vi "PH_PILS.vis extExpKnob.vi"(0 "i ref in":refnum<vi>, 5 "error IO":errorcluster) -> (14 "i ref out":refnum<vi>, 19 "error out":errorcluster)   [LabVIEW 2014, in "PH_PILS.lvlib"]
uses:
  PH_PILS.lvlib
  PH_Basics/PH_Common/PH_Common.lvlib
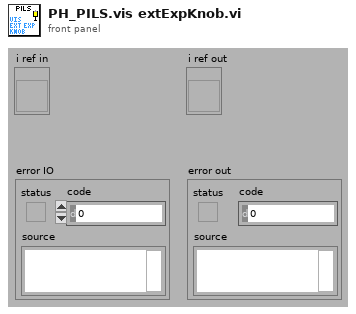
[diagram p1: front panel]
types:
  T1 = typedef "PH_PILS.lvlib/PH_PILS.i attribute.ctl" = cluster{"Boolean":cluster{"GUI Ref":refnum<vi>, "Status":i32}[], "GUI Refs Exp. Shutters":cluster{"1":refnum<vi>, "2":refnum<vi>, "3":refnum<vi>, "4":refnum<vi>}, "Tristate2Run GUI Refs":refnum<vi>[], "EO-Likes":cluster{"GUI Ref":refnum<vi>, "Status":i32}[], "Operation Mode":cluster{"Operation Mode":T2, "GUI":cluster{"Ref State":refnum<vi>, "Ref":refnum<vi>}, "Servicemode":cluster{"Tagname":string, "Status":i32}, "Labormode":cluster{"Tagname":string, "Status":i32}, "Searchmode":cluster{"Tagname":string, "Status":i32}, "Shotmode":cluster{"Tagname":string, "Status":i32}}, "Submode":cluster{"Submode":T3, "GUI":cluster{"Ref State":refnum<vi>, "Ref":refnum<vi>}, "Submode":cluster{"Tagname":string, "Status":i32}}, "Experiment":cluster{"Experiment":enum16{"unknown", "intern", "4 (Z6)", "3", "2", "1"}, "GUI":cluster{"Ref State":refnum<vi>, "Ref":refnum<vi>}, "intern":cluster{"Tagname":string, "Status":i32}, "Exp 4":cluster{"Tagname":string, "Status":i32}, "Exp 3":cluster{"Tagname":string, "Status":i32}, "Exp 2":cluster{"Tagname":string, "Status":i32}, "Exp 1":cluster{"Tagname":string, "Status":i32}}, "TristateNormal":cluster{"GUI Ref":refnum<vi>, "Status":i32}[], "Door Tags":cluster{"GUI Ref":refnum<vi>, "Status":i32}[], "GUIlessTags":cluster{"Name":string, "Status":i32}[], "Beamline GUI Refs":refnum<vi>[], "Special Boolean":cluster{"GUI Ref":refnum<vi>, "Status":i32}[], "Laserpower":cluster{"GUI Ref":refnum<vi>, "Status":i32}[], "Shutter":cluster{"GUI Ref":refnum<vi>, "Status":i32}[], "Tristate EO Like":cluster{"GUI Ref":refnum<vi>, "Status":i32}[], "PP":cluster{"GUI Ref":refnum<vi>, "Status":i32, "Head Ref":refnum<vi>, "Slider Ref":refnum<vi>}[], "Switch Knobs":cluster{"GUI Ref":refnum<vi>, "Status":i32}[], "Latch Knob GUI Refs":refnum<vi>[], "FailureCounter":i32, "Enabled Status":cluster{"Laser":i32, "PreAmp":i32, "MainAmp":i32}, "Mercury":refnum<vi>, "Instance Rods":string, "Logfile":path, "Beckhoff-Instance Internal":string, "Beckhoff-Instance External":string, "Enabling Rights":cluster{"Name":string, "Password":string, "PA?":bool, "MA?":bool, "Exp?":bool}[]}
  T2 = typedef "PH_PILS.lvlib/PH_PILS.Operation Mode.ctl" = enum16{"unknown", "Service", "Labor", "Search", "Shot"}
  T3 = typedef "PH_PILS.lvlib/PH_PILS.Submode.ctl" = enum16{"unknown", "HV-Normal", "HV-Test"}
  T4 = enum16{"unknown", "intern", "4 (Z6)", "3", "2", "1"}
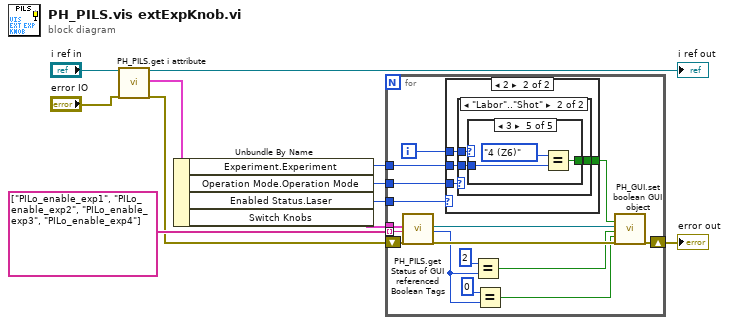
[diagram p0: block diagram]
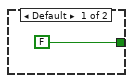
[diagram p2: hidden frame]
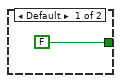
[diagram p3: hidden frame]
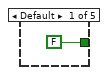
[diagram p4: hidden frame]
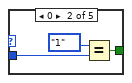
[diagram p5: hidden frame]
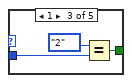
[diagram p6: hidden frame]
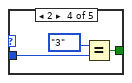
[diagram p7: hidden frame]
diagram:
  n1 = call "PH_PILS.get i attribute.vi"("i ref in"="i ref in", "error in (no error)"="error IO") -> ("i ref out"=→"i ref out":refnum<vi>, "i attribute"=w6:T1, "error out"=w1:errorcluster)  [unwired: 15 in]
  n2 = Unbundle By Name(w6) -> ("Experiment.Experiment"=w5:T4, "Operation Mode.Operation Mode"=w4:T2, "Enabled Status.Laser"=w3:i32, "Switch Knobs"=w7:cluster{"GUI Ref":refnum<vi>, "Status":i32}[])
  n3 = for {
    tunnel: w7 -> [w27]
    tunnel: string[] ["PILo_enable_exp1", "PILo_enable_exp2", "PILo_enable_exp3", "PILo_enable_exp4"] -> [w20] mode=indexing
    tunnel: w5 -> [w18]
    tunnel: w4 -> [w16]
    tunnel: w3 -> [w12]
    shift-right: [w24] -> w11
    shift-left: w1 -> [w23]
    i -> [w19]
    n4 = call "PH_PILS.get Status of GUI referenced Boolean Tags.vi"("Tags"=w27, "Tagname"=w20, "error in"=w23) -> ("GUI Ref"=w25:refnum<vi>, "Status"=w15:i32, "error out"=w26:errorcluster)  [unwired: 13 in, 1 out]
    n5 = case shown="2" w12 {
      tunnel: w19 -> [_ w32]
      tunnel: w18 -> [_ w31]
      tunnel: [FALSE w30] -> w17
      tunnel: w16 -> [_ w29]
      frame Default {
      }
      frame 2 {
        n6 = case shown="\"Labor\"..\"Shot\"" w29 {
          tunnel: w32 -> [_ w36]
          tunnel: w31 -> [_ w35]
          tunnel: [FALSE w34] -> w30
          frame Default {
          }
          frame "Labor".."Shot" {
            n7 = case shown="3" w36 {
              tunnel: w35 -> [_ w39 w42 w45 w48]
              tunnel: [FALSE w38 w41 w44 w47] -> w34
              frame Default {
              }
              frame 0 {
                n8 = Equal?(x=T4."1" ("Experiment.Experiment"), y=w39) -> (x = y?=w38:bool)
              }
              frame 1 {
                n9 = Equal?(x=T4."2" ("Experiment.Experiment"), y=w42) -> (x = y?=w41:bool)
              }
              frame 2 {
                n10 = Equal?(x=T4."3" ("Experiment.Experiment"), y=w45) -> (x = y?=w44:bool)
              }
              frame 3 {
                n11 = Equal?(x=T4."4 (Z6)" ("Experiment.Experiment"), y=w48) -> (x = y?=w47:bool)
              }
            }
          }
        }
      }
    }
    n12 = Equal?(x=2, y=w15) -> (x = y?=w21:bool)
    n13 = Equal?(x=0, y=w15) -> (x = y?=w14:bool)
    n14 = call "PH_GUI.set boolean GUI object.vi"("Visible (true)"=w17, "Boolean Knob GUI Ref"=w25, "Value"=w21, "Blinking? (false)"=w14, "error in (no error)"=w26) -> ("error out"=w24:errorcluster)  [unwired: 14 in]
  }
  "error out" <- w11
